vi "simplePID core_FXP_integralsatfixed.vi"(0 "errors":T1, 1 "reset? (F)":bool, 7 "manual control":T6, 11 "state in":T3, 12 "gains":T4, 13 "output range":T5={"output high (Inf)"=2047.99609375, "output low (-Inf)"=-2048.0}) -> (4 "output":fxp<+/-,20,12>, 6 "error":fxp<+/-,16,10>, 8 "actions":T2, 15 "state out":T3)   [LabVIEW 2020]
uses:
  Typedef/niFpgaPID_ManualControl_FXP.ctl
  Typedef/niFpgaPID_OutputRange_FXP.ctl
  Typedef/niFpgaPID_PIDGains_FXP.ctl
  Typedef/niFpgaPID_PIDState_FXP.ctl
  Typedef/niFpgaPID_PIDActions_FXP.ctl
  Typedef/niFpgaPID_PIDErrors_FXP.ctl
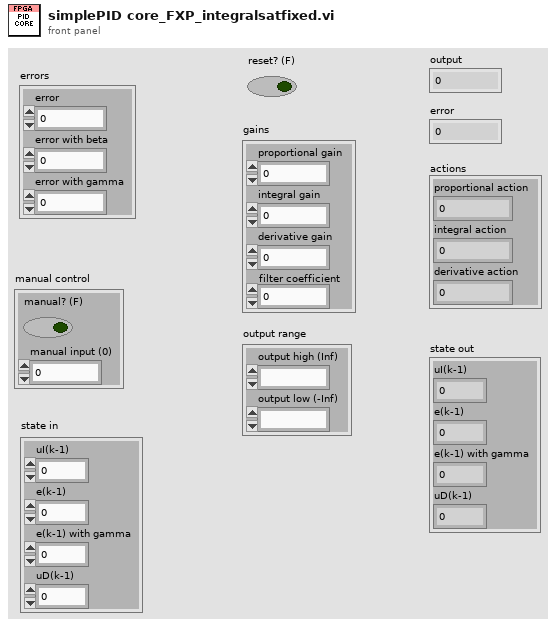
[diagram p1: front panel]
types:
  T1 = typedef "niFpgaPID_PIDErrors_FXP.ctl" = cluster{"error":fxp<+/-,16,10>, "error with beta":fxp<+/-,16,10>, "error with gamma":fxp<+/-,16,10>}
  T2 = typedef "niFpgaPID_PIDActions_FXP.ctl" = cluster{"proportional action":fxp<+/-,20,12>, "integral action":fxp<+/-,20,12>, "derivative action":fxp<+/-,20,12>}
  T3 = typedef "niFpgaPID_PIDState_FXP.ctl" = cluster{"uI(k-1)":fxp<+/-,20,12>, "e(k-1)":fxp<+/-,16,10>, "e(k-1) with gamma":fxp<+/-,16,10>, "uD(k-1)":fxp<+/-,20,12>}
  T4 = typedef "niFpgaPID_PIDGains_FXP.ctl" = cluster{"proportional gain":fxp<+/-,17,4>, "integral gain":fxp<+/-,16,3>, "derivative gain":fxp<+/-,16,3>, "filter coefficient":fxp<+/-,17,4>}
  T5 = typedef "niFpgaPID_OutputRange_FXP.ctl" = cluster{"output high (Inf)":fxp<+/-,20,12>, "output low (-Inf)":fxp<+/-,20,12>}
  T6 = typedef "niFpgaPID_ManualControl_FXP.ctl" = cluster{"manual? (F)":bool, "manual input (0)":fxp<+/-,20,12>}
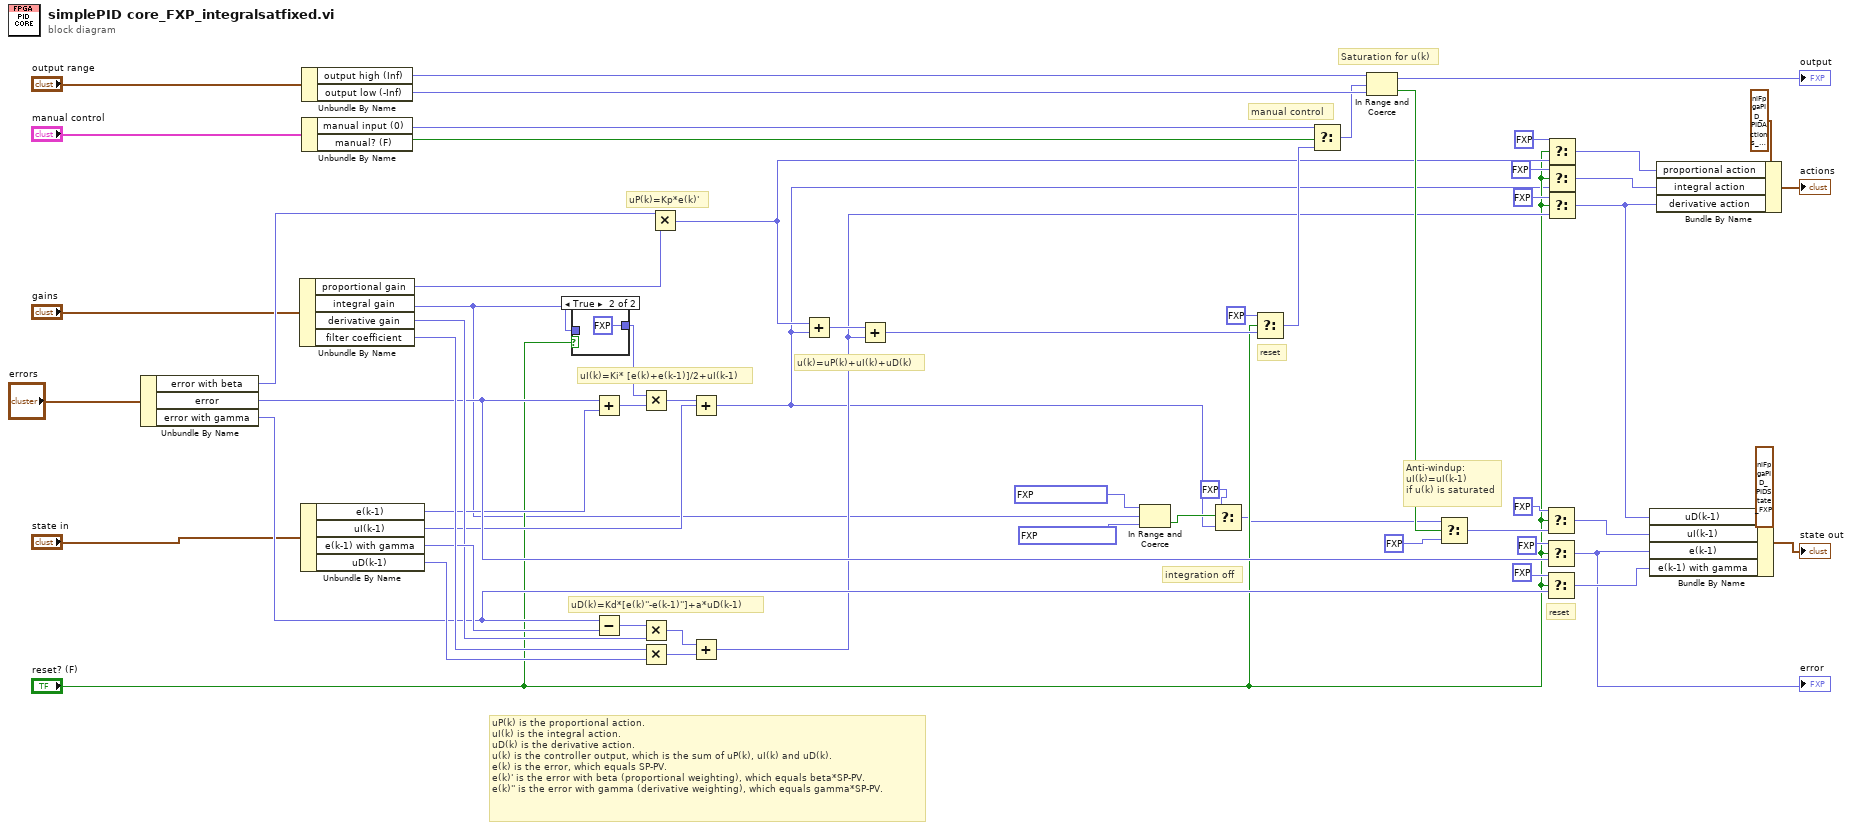
[diagram p0: block diagram]
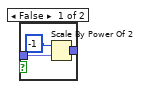
[diagram p2: hidden frame]
diagram:
  # "uP(k) is the proportional action.\nuI(k) is the integral action.\nuD(k) is the derivative action.\nu(k) is the controller output, which is the sum of uP(k), uI(k) and uD(k).\ne(k) is the error, which equals SP-PV.\ne(k)' is the error with beta (proportional weighting), which equals beta*SP-PV.\ne(k)'' is the error with gamma (derivative weighting), which equals gamma*SP-PV."
  # "manual control"
  # "reset"
  # "reset"
  # "integration off"
  # "u(k)=uP(k)+uI(k)+uD(k)"
  # "uI(k)=Ki* [e(k)+e(k-1)]/2+uI(k-1)"
  # "uD(k)=Kd*[e(k)''-e(k-1)'']+a*uD(k-1)"
  # "uP(k)=Kp*e(k)'"
  # "Anti-windup:\nuI(k)=uI(k-1) \nif u(k) is saturated"
  # "Saturation for u(k)"
  n1 = Unbundle By Name("errors") -> ("error with beta"=w48:fxp<+/-,16,10>, "error"=w36:fxp<+/-,16,10>, "error with gamma"=w35:fxp<+/-,16,10>)
  n2 = Unbundle By Name("gains") -> ("proportional gain"=w49:fxp<+/-,17,4>, "integral gain"=w6:fxp<+/-,16,3>, "derivative gain"=w44:fxp<+/-,16,3>, "filter coefficient"=w54:fxp<+/-,17,4>)
  n3 = Unbundle By Name("state in") -> ("e(k-1)"=w27:fxp<+/-,16,10>, "uI(k-1)"=w26:fxp<+/-,20,12>, "e(k-1) with gamma"=w47:fxp<+/-,16,10>, "uD(k-1)"=w53:fxp<+/-,20,12>)
  n4 = Unbundle By Name("output range") -> ("output high (Inf)"=w59:fxp<+/-,20,12>, "output low (-Inf)"=w58:fxp<+/-,20,12>)
  n5 = Unbundle By Name("manual control") -> ("manual input (0)"=w43:fxp<+/-,20,12>, "manual? (F)"=w42:bool)
  n6 = case shown="True" "reset? (F)" {
    tunnel: [w62 fxp<+/-,16,3> 0.0] -> w45
    tunnel: w6 -> [w61 _]
    frame False {
      n7 = Scale By Power Of 2(n=i16 -1, x=w61) -> (x*2^n=w62:fxp<+/-,16,3>)
    }
    frame True {
    }
  }
  n8 = Add(x=w36, y=w27) -> (x+y=w46:fxp<+/-,19,12>)
  n9 = Subtract(x=w35, y=w47) -> (x-y=w52:fxp<+/-,18,11>)
  n10 = Multiply(x=w45, y=w46) -> (x*y=w56:fxp<+/-,20,12>)
  n11 = Multiply(x=w52, y=w44) -> (x*y=w51:fxp<+/-,20,12>)
  n12 = Multiply(x=w54, y=w53) -> (x*y=w50:fxp<+/-,20,12>)
  n13 = Multiply(x=w48, y=w49) -> (x*y=w29:fxp<+/-,20,12>)
  n14 = Add(x=w56, y=w26) -> (x+y=w2:fxp<+/-,20,12>)
  n15 = Add(x=w51, y=w50) -> (x+y=w32:fxp<+/-,20,12>)
  n16 = Add(x=w29, y=w2) -> (x+y=w55:fxp<+/-,20,12>)
  n17 = Add(x=w55, y=w32) -> (x+y=w17:fxp<+/-,20,12>)
  n18 = In Range and Coerce(upper limit=fxp<+/-,16,3> 0.0001220703125, x=w6, lower limit=fxp<+/-,16,3> -0.0001220703125) -> (In Range?=w3:bool)  [unwired: 1 out]
  n19 = Select(t=fxp<+/-,20,12> 0.0, s=w3, f=w2) -> (s? t:f=w8:fxp<+/-,20,12>)
  n20 = Select(t=fxp<+/-,20,12> 0.0, s="reset? (F)", f=w17) -> (s? t:f=w40:fxp<+/-,20,12>)
  n21 = Select(t=w43, s=w42, f=w40) -> (s? t:f=w57:fxp<+/-,20,12>)
  n22 = In Range and Coerce(upper limit=w59, x=w57, lower limit=w58) -> (coerced(x)=→"output":fxp<+/-,20,12>, In Range?=w60:bool)
  n23 = Select(t=w8, s=w60, f=fxp<+/-,20,12> 0.0) -> (s? t:f=w37:fxp<+/-,20,12>)
  n24 = Select(t=fxp<+/-,20,12> 0.0, s="reset? (F)", f=w37) -> (s? t:f=w38:fxp<+/-,20,12>)
  n25 = Select(t=fxp<+/-,16,10> 0.0, s="reset? (F)", f=w36) -> (s? t:f=w18:fxp<+/-,16,10>)
  "error" <- w18
  n26 = Select(t=fxp<+/-,16,10> 0.0, s="reset? (F)", f=w35) -> (s? t:f=w34:fxp<+/-,16,10>)
  n27 = Select(t=fxp<+/-,20,12> 0.0, s="reset? (F)", f=w29) -> (s? t:f=w30:fxp<+/-,20,12>)
  n28 = Select(t=fxp<+/-,20,12> 0.0, s="reset? (F)", f=w2) -> (s? t:f=w28:fxp<+/-,20,12>)
  n29 = Select(t=fxp<+/-,20,12> 0.0, s="reset? (F)", f=w32) -> (s? t:f=w31:fxp<+/-,20,12>)
  n30 = Bundle By Name(cluster=T3 {"uI(k-1)"=0.0, "e(k-1)"=0.0, "e(k-1) with gamma"=0.0, "uD(k-1)"=0.0} ("state"), "uD(k-1)"=w31, "uI(k-1)"=w38, "e(k-1)"=w18, "e(k-1) with gamma"=w34) -> (→"state out":T3)
  n31 = Bundle By Name(cluster=T2 {"proportional action"=0.0, "integral action"=0.0, "derivative action"=0.0} ("actions"), "proportional action"=w30, "integral action"=w28, "derivative action"=w31) -> (→"actions":T2)
